vi "Read serializble from table.vi"(7 "serializers":refnum<class "BlueSerializer.lvclass">[](array[class]), 8 "error in":errorcluster, 11 "Table ref in":refnum<vi>) -> (0 "error out":errorcluster, 2 "serializable texts":string[](array[string]), 3 "Table ref out":refnum<vi>)   [LabVIEW 2019, in "Sports Unit Tests.lvclass"]
uses:
  Sports Unit Tests.lvclass
  <userlib>/Blue Origin/BlueSerialization/BlueSerializer/BlueSerializer.lvclass
  <vilib>/Utility/error.llb/Error Cluster From Error Code.vi
  <vilib>/ErrorRing/Error Ring.xnode
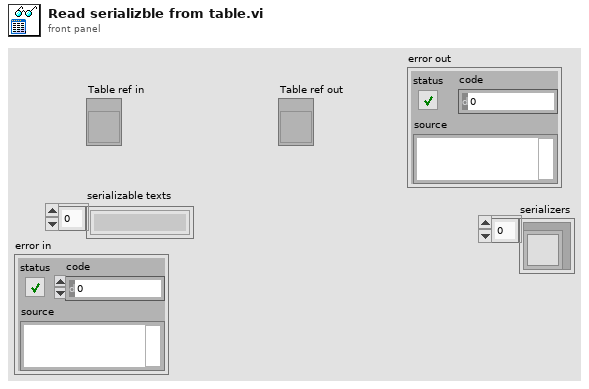
[diagram p1: front panel]
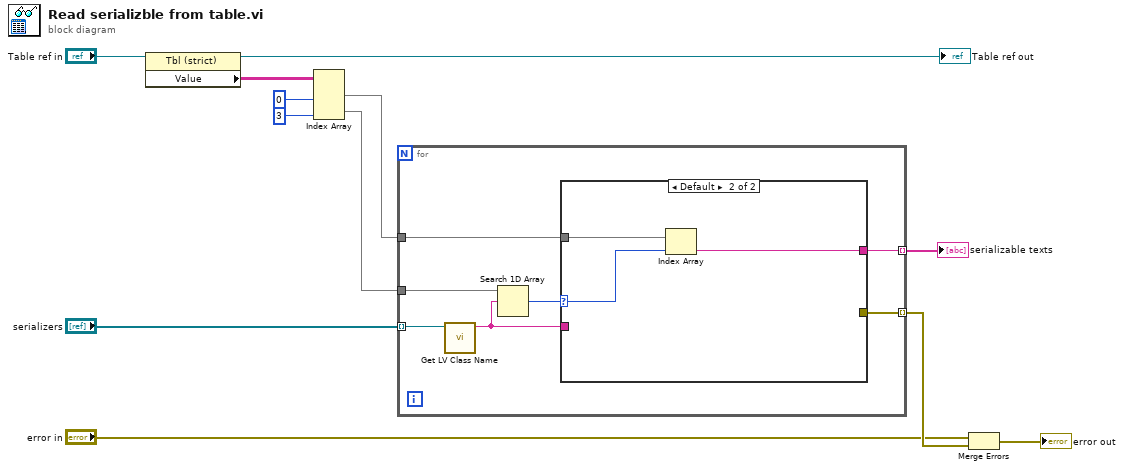
[diagram p0: block diagram]
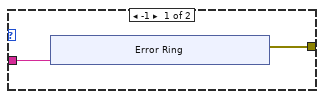
[diagram p2: hidden frame]
diagram:
  n1 = property class="Tbl (strict)"(reference="Table ref in") -> (reference out=→"Table ref out":refnum<vi>, "Value"=w10:string[][])  [unwired: 1 in, 1 out]
  n2 = Index Array(array=w10, index (col) #1=0 ("disabled index (col)"), index (col) #2=3 ("index (col)")) -> (element #1=w5:string[], element #2=w6:string[])  [unwired: 2 in]
  n3 = for {
    tunnel: "serializers" -> [w19] mode=indexing
    tunnel: w6 -> [w18]
    tunnel: w5 -> [w17]
    tunnel: [w15] -> w4 mode=indexing
    tunnel: [w13] -> w3 mode=indexing
    n4 = call <vilib>:"Get LV Class Name.vi"("object"=w19) -> ("class name"=w14:string)  [unwired: 9 in, 1 out]
    n5 = Search 1D Array(1D array=w18, element=w14) -> (index of element=w16:i32)  [unwired: 1 in]
    n6 = case shown="Default" w16 {
      selector: w16 -> [_ w30]
      tunnel: w17 -> [_ w31]
      tunnel: [_ w29] -> w15
      tunnel: w14 -> [w21 _]
      tunnel: [w20 _] -> w13
      frame -1 {
        n7 = xnode "Error Ring"("parameter 0"=w21) -> ("error out"=w20:errorcluster)
      }
      frame Default {
        n8 = Index Array(array=w31, index=w30) -> (element=w29:string)
      }
    }
  }
  "serializable texts" <- w4
  n9 = Merge Errors("error in", w3) -> (→"error out":errorcluster)
